vi "Get Kasli IP.vi"(8 "error in (no error)":errorcluster, 11 "Kasli Listener in":refnum<class "Kasli Listener.lvclass">) -> (0 "error out":errorcluster, 3 "Kasli Listener out":refnum<class "Kasli Listener.lvclass">)   [LabVIEW 2020, in "Kasli Listener and Writer.lvlib" / "Kasli Listener.lvclass"]
uses:
  Kasli Listener.lvclass
  C:/Users/marco/Documents/GitHub_Lab/TALOS/talos/Ancestor/Ancestor/Ancestor.lvclass
  C:/Users/marco/Documents/GitHub_Lab/TALOS/talos/Internal uServices/System uServices/TCP Listener/TCP Listener/TCP Listener.lvclass
  Ancestor/Ancestor/Ancestor.lvclass/Ancestor.ctl
  Ancestor/Ancestor/Read ID.vi
  Support VIs/Generate Error.vi
  FGV/Error Memory/Get Error Description.vi
  Support VIs/Get PC name.vi
  Support VIs/Get Class Name.vi
  <vilib>/Utility/error.llb/Clear Errors.vi
  FGV/Error Memory/Error Memory Core.vi
  <vilib>/AdvancedString/Delimited String to 1D String Array.vi
  Support VIs/Circus Root Path.vi
  FGV/Error Memory/Error Crt Lvl checker.vi
  FGV/Error Memory/Error Memory Core.vi/40c8088d-b597-4017-91af-faa98e00292e.vi
  FGV/Error Memory/Error Memory Core.vi/d4a3ab98-063c-4e44-b43d-fbdcfe6c2be2.vi
  Support VIs/Global Memory.vi
  <vilib>/Utility/LVClass/Get LV Class Name.vi
  Support VIs/Is in Packed Library.vi
  Support VIs/TALOS Root path.vi
  Support VIs/Read CSV worksheet.vi
  Support VIs/Global Constants.vi
  <vilib>/Utility/error.llb/General Error Handler.vi
  Ancestor/Ancestor/Ancestor.lvclass
  <vilib>/Comparison/Equal/Equal Functor/Equal Functor.lvclass
  Kasli Listener.lvclass/Kasli Listener.ctl
  TALOS.lvlib
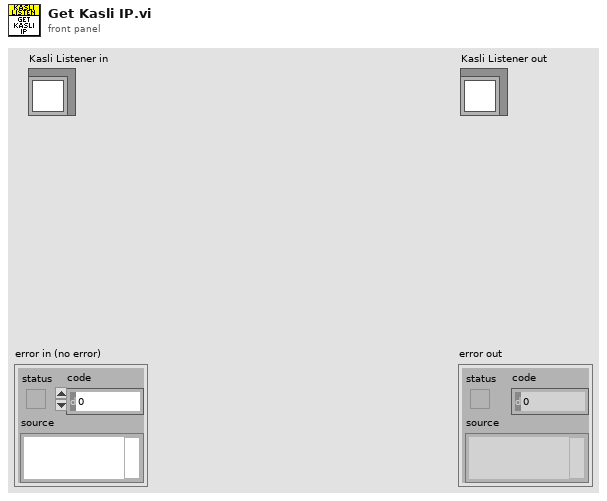
[diagram p1: front panel]
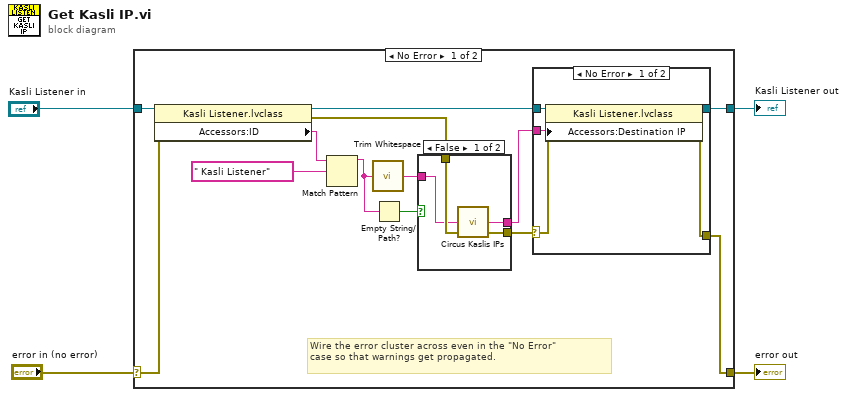
[diagram p0: block diagram]
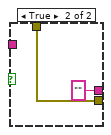
[diagram p3: hidden frame]
diagram:
  n1 = case shown="No Error" "error in (no error)" {
    selector: "error in (no error)" -> [w9 w32]
    tunnel: [w5 w32] -> w3
    tunnel: [w8 w31] -> w1
    tunnel: "Kasli Listener in" -> [w17 w31]
    frame No Error {
      # "Wire the error cluster across even in the \"No Error\"\ncase so that warnings get propagated."
      n2 = property class="Kasli Listener.lvclass"(reference=w17, error in=w9) -> (reference out=w16:refnum<class "Kasli Listener.lvclass">, error out=w10:errorcluster, "Accessors:ID"=w15:string)
      n3 = Match Pattern(string=w15, regular expression=" Kasli Listener") -> (before substring=w11:string)  [unwired: 1 in, 3 out]
      n4 = call <vilib>:"Trim Whitespace.vi"("string"=w11) -> ("trimmed string"=w12:string)  [unwired: 1 in]
      n5 = Empty String/Path?(string/path=w11) -> (empty?=w13:bool)
      n6 = case shown="False" w13 {
        tunnel: w12 -> [w27 _]
        tunnel: [w26 "" ("IP")] -> w7
        tunnel: [w25 w29] -> w6
        tunnel: w10 -> [w28 w29]
        frame False {
          n7 = call "Circus Kaslis IPs.vi"("error in (no error)"=w28, "ID"=w27) -> ("error out"=w25:errorcluster, "IP"=w26:string)  [unwired: 2 in]
        }
        frame True {
        }
      }
      n8 = case shown="No Error" w6 {
        selector: w6 -> [w22 w23]
        tunnel: w16 -> [w21 w24]
        tunnel: [w20 w24] -> w8
        tunnel: w7 -> [w19 _]
        tunnel: [w18 w23] -> w5
        frame No Error {
          n9 = property class="Kasli Listener.lvclass"(reference=w21, error in=w22, "Accessors:Destination IP"=w19) -> (reference out=w20:refnum<class "Kasli Listener.lvclass">, error out=w18:errorcluster)
        }
        frame Error {
        }
      }
    }
    frame Error {
    }
  }
  "error out" <- w3
  "Kasli Listener out" <- w1
